vi "Daqmx junk.vi"   [LabVIEW 2015]
uses:
  <vilib>/DAQmx/configure/timing.llb/DAQmx Timing (Sample Clock).vi
  <vilib>/DAQmx/write.llb/DAQmx Write (Analog 1D Wfm NChan NSamp).vi
  <vilib>/DAQmx/create/channels.llb/DAQmx Create Channel (AI-Voltage-Basic).vi
  <vilib>/DAQmx/create/channels.llb/DAQmx Create Channel (AO-Voltage-Basic).vi
  <vilib>/DAQmx/write.llb/DAQmx Write (Digital 1D Wfm NChan NSamp).vi
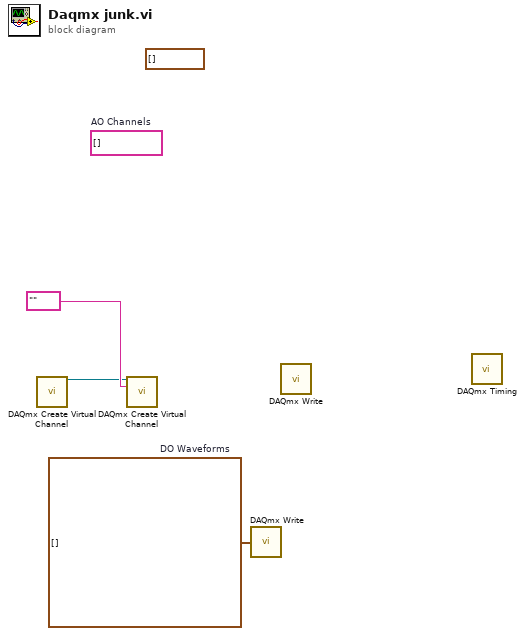
[diagram p0: block diagram]
diagram:
  w1 = digitalwaveform[] []  # DO Waveforms
  (unwired) waveform(dbl)[] [] ("AO Waveforms")
  (unwired) tag[] []  # AO Channels
  n1 = call-poly <vilib>:"DAQmx Create Virtual Channel.vi"() -> ("task out"=w3:refnum<k21>, "physical channels"=w5:tag)  [unwired: 13 in, 1 out]
  n2 = call-poly <vilib>:"DAQmx Create Virtual Channel.vi"("task in"=w3, "physical channels"=tag "") -> ()  [unwired: 12 in, 2 out]
  n3 = call-poly <vilib>:"DAQmx Write.vi"("data"=w1) -> ()  [unwired: 12 in, 3 out]
  n4 = call-poly <vilib>:"DAQmx Write.vi"() -> ("task/channels in"=w6:refnum<k21>, "data"=w2:waveform(dbl)[])  [unwired: 11 in, 3 out]
  n5 = call-poly <vilib>:"DAQmx Timing.vi"() -> ()  [unwired: 14 in, 2 out]
